vi "Auton-MoveToAuto.vi"() -> (2 "Boolean":bool)   [LabVIEW 2014]
uses:
  <vilib>/Rock Robotics/WPI/RobotDrive/WPI_RobotDriveGetSetRefNum.vi
  <vilib>/Rock Robotics/WPI/RobotDrive/WPI_RobotDriveArcadeDrive_Standard(NoSaturation).vi
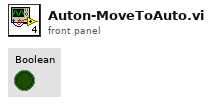
[diagram p1: front panel]
types:
  T1 = typedef "WPI_GyroDevRef.ctl" = cluster{"DevStatus":errorcluster, "Analog Module":T2, "Analog Channel":T3, "Offset":dbl, "Gain (VoltsPerDegree/Second)":dbl}
  T2 = typedef "FPGA_TypedefAnalogModule.ctl" = enum16{"Controller 1"}
  T3 = typedef "FPGA_AIChannel.ctl" = enum8{"AI 0", "AI 1", "AI 2", "AI 3", "AI MXP 0", "AI MXP 1", "AI MXP 2", "AI MXP 3", "Invalid"}
  T4 = typedef "WPI_RobotDriveDevRef.ctl" = cluster{"DevStatus":errorcluster, "Motors[]":T5[], "Square Inputs":bool, "Max Output":dbl}
  T5 = typedef "WPI_MotorControlDeviceRef.ctl" = cluster{"DeviceStatus":errorcluster, "Type":T6, "PWM":cluster{"Controller":T7, "PWM Channel":T8, "DeadBand":T9}, "CAN":cluster{"Device Number":u8, "Control Mode":T10, "Semaphore":T11, "Max Vout":dbl, "TalonSRX Control Mode":T12}, "Invert":bool, "TransformRef":T13, "InvTransformRef":T13}
  T6 = typedef "WPI_MotorControlType.ctl" = enum16{"PWM", "CAN", "CANTalonSRX"}
  T7 = typedef "FPGA_TypedefDigitalModule.ctl" = enum16{"Controller 1"}
  T8 = typedef "FPGA_DIOPWMChannel.ctl" = enum8{"PWM 0", "PWM 1", "PWM 2", "PWM 3", "PWM 4", "PWM 5", "PWM 6", "PWM 7", "PWM 8", "PWM 9", "PWM MXP 0", "PWM MXP 1", "PWM MXP 2", "PWM MXP 3", "PWM MXP 4", "PWM MXP 5", "PWM MXP 6", "PWM MXP 7", "PWM MXP 8", "PWM MXP 9", "Invalid"}
  T9 = typedef "WPI_PWMDeadband.ctl" = cluster{"Name":string, "maxPositivePwm":i32, "minPositivePwm":i32, "centerPwm":i32, "maxNegativePwm":i32, "minNegativePwm":i32, "angularRange":u16}
  T10 = typedef "WPI_CANJaguar_ControlMode.ctl" = enum8{"Percent VBus", "Current", "Speed", "Position", "Voltage"}
  T11 = typedef "Semaphore RefNum" = refnum<k1>
  T12 = typedef "WPI_CANTalonSRX_APIControlMode.ctl" = enum8{"Percent VBus", "Speed", "Position", "Slave", "Unchanged / Invalid"}
  T13 = typedef "WPI_PWMTransform_ConPane.ctl" = refnum<vi>
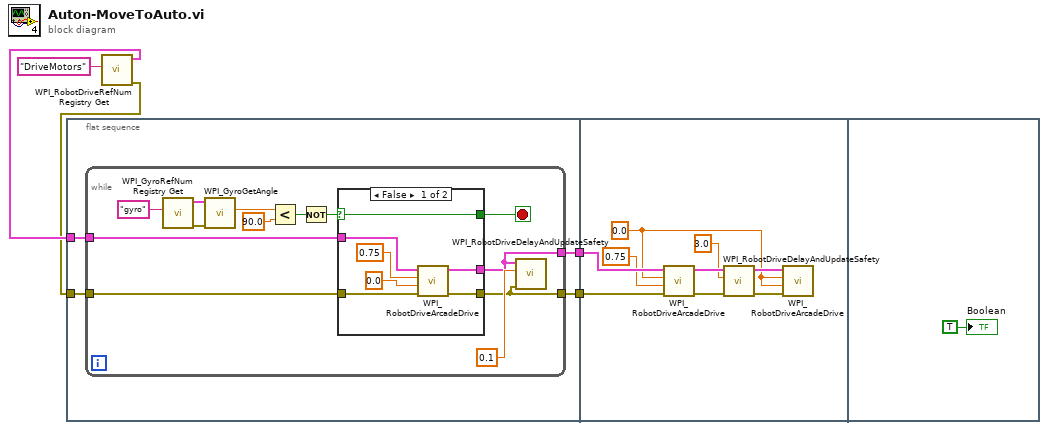
[diagram p0: block diagram]
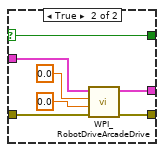
[diagram p2: hidden frame]
diagram:
  n1 = flat-sequence {
    tunnel: w4 -> [w9]
    tunnel: w3 -> [w8]
    tunnel: [w7] -> w2
    tunnel: [w6] -> w1
    tunnel: w2 -> [w45]
    tunnel: w1 -> [w44]
    frame #0 {
      n2 = while {
        tunnel: w9 -> [w13]
        tunnel: w8 -> [w12]
        tunnel: [w11] -> w7
        tunnel: [w10] -> w6
        stop <- w14 stop-if-true
        n3 = call <vilib>:"WPI_GyroRefNum Registry Get.vi"("refnum name"="gyro") -> ("error out"=w21:errorcluster, "GyroDevRef"=w20:T1)  [unwired: 9 in]
        n4 = call <vilib>:"WPI_GyroGetAngle.vi"("error in (no error)"=w21, "GyroDevRef"=w20) -> ("Angle"=w18:dbl)  [unwired: 6 in, 3 out]
        n5 = Less?(x=w18, y=90.0) -> (x < y?=w15:bool)
        n6 = Not(x=w15) -> (.not. x?=w16:bool)
        n7 = case shown="False" w16 {
          selector: w16 -> [w23 w30]
          tunnel: w13 -> [w27 w35]
          tunnel: w12 -> [w26 w34]
          tunnel: [w25 w33] -> w11
          tunnel: [w24 w32] -> w10
          tunnel: [w23 w30] -> w14
          frame False {
            n8 = call-poly <vilib>:"WPI_RobotDriveArcadeDrive.vi"("error in (no error)"=w26, "Y axis value"=0.0, "X axis value"=0.75, "RobotDriveDevRef"=w27) -> ("error out"=w24:errorcluster, "RobotDriveDevRef"=w25:T4)  [unwired: 5 in, 1 out]
          }
          frame True {
            n9 = call-poly <vilib>:"WPI_RobotDriveArcadeDrive.vi"("error in (no error)"=w34, "Y axis value"=0.0, "X axis value"=0.0, "RobotDriveDevRef"=w35) -> ("error out"=w32:errorcluster, "RobotDriveDevRef"=w33:T4)  [unwired: 5 in, 1 out]
          }
        }
        n10 = call <vilib>:"WPI_RobotDriveDelayAndUpdateSafety.vi"("error in (no error)"=w10, "Delay (s)"=0.1 ("dt (s)"), "RobotDriveDevRef"=w11) -> ()  [unwired: 7 in, 2 out]
      }
    }
    frame #1 {
      w37 = 0.0 ("X axis value")
      n11 = call-poly <vilib>:"WPI_RobotDriveArcadeDrive.vi"("error in (no error)"=w44, "Y axis value"=0.75, "X axis value"=w37, "RobotDriveDevRef"=w45) -> ("error out"=w41:errorcluster, "RobotDriveDevRef"=w42:T4)  [unwired: 5 in, 1 out]
      n12 = call <vilib>:"WPI_RobotDriveDelayAndUpdateSafety.vi"("error in (no error)"=w41, "Delay (s)"=3.0, "RobotDriveDevRef"=w42) -> ("error out"=w39:errorcluster, "RobotDriveDevRef 2"=w38:T4)  [unwired: 7 in]
      n13 = call-poly <vilib>:"WPI_RobotDriveArcadeDrive.vi"("error in (no error)"=w39, "Y axis value"=w37, "X axis value"=w37, "RobotDriveDevRef"=w38) -> ()  [unwired: 5 in, 3 out]
    }
    frame #2 {
      "Boolean" <- TRUE ("Boolean")
    }
  }
  n14 = call <vilib>:"WPI_RobotDriveRefNum Registry Get.vi"("refnum name"="DriveMotors") -> ("error out"=w3:errorcluster, "RobotDriveDevRef"=w4:T4)  [unwired: 9 in]
